vi "wave2xwav.vi"(4 "waveform":waveform(dbl)) -> (1 "xwave":T1={"attributes"=variant, "X"={"start"=0.0, "delta"=0.0, "units"="index", "dim"="au"}, "Y"={"data"=[], "units"="au"}})   [LabVIEW 2015]
uses:
  xwav.ctl
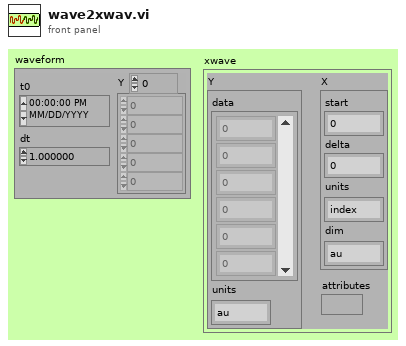
[diagram p1: front panel]
types:
  T1 = typedef "xwav.ctl" = cluster{"attributes":variant, "X":cluster{"start":dbl, "delta":dbl, "units":string, "dim":string}, "Y":cluster{"data":dbl[], "units":string}}
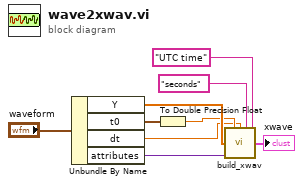
[diagram p0: block diagram]
diagram:
  n1 = Unbundle By Name("waveform") -> ("Y"=w7:dbl[], "t0"=w6:timestamp, "dt"=w4:dbl, "attributes"=w3:variant)
  n2 = To Double Precision Float(number=w6) -> (double precision float=w5:dbl)
  n3 = call "build_xwav.vi"("x0 (0)"=w5, "dx (1)"=w4, "x units (index)"="seconds", "x dimention (x)"="UTC time" ("x units"), "Y"=w7, "attributes"=w3) -> ("xwave"=→"xwave":T1)  [unwired: 9 in]
